vi "007 gràfic temperatura 3 darrers valors.vi"() -> ()   [LabVIEW 2019]
panel:
  out "Waveform Chart":cluster{"temp":dbl, dbl, dbl}(graph)
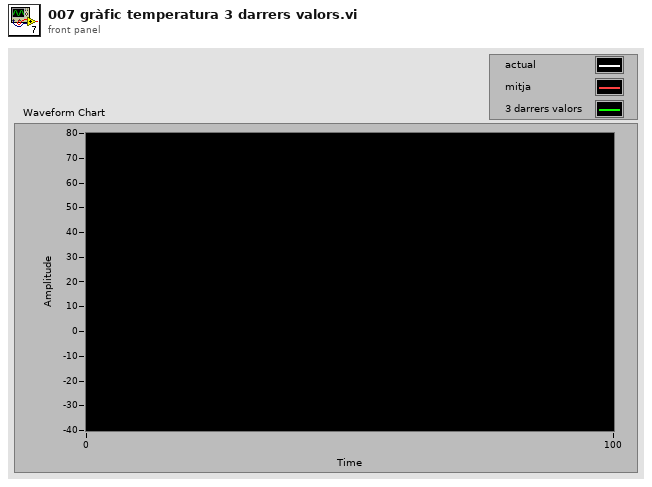
[diagram p1: front panel]
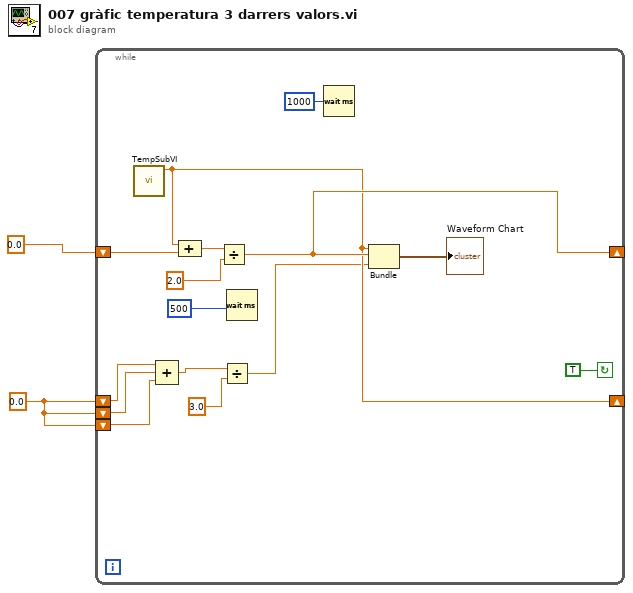
[diagram p0: block diagram]
diagram:
  w1 = 0.0 ("temp")
  n1 = while {
    shift-right: [w11] -> _
    shift-left: 0.0 -> [w12]
    shift-right: [w10] -> _
    shift-left: w1 -> [w9]
    shift-left: w1 -> [w8]
    shift-left: w1 -> [w7]
    stop <- TRUE continue-if-true
    n2 = call "TempSubVI.vi"() -> ("temp"=w10:dbl)  [unwired: 11 in]
    n3 = Compound Arithmetic op=ADD(w9, w8, w7) -> (w6:dbl)
    n4 = Compound Arithmetic op=ADD(w10, w12) -> (w14:dbl)
    n5 = Divide(x=w14, y=2.0) -> (x/y=w11:dbl)
    n6 = Divide(x=w6, y=3.0) -> (x/y=w4:dbl)
    n7 = Wait (ms)(milliseconds to wait=500) -> ()  [unwired: 1 out]
    n8 = Wait (ms)(milliseconds to wait=u32 1000) -> ()  [unwired: 1 out]
    n9 = Bundle("temp"=w10, w11, w4) -> (→"Waveform Chart":cluster{"temp":dbl, dbl, dbl})  [unwired: 1 in]
  }
